vi "FAR_IR_CM_to_NEAR_IR_NM.vi"(11 "Far IR / cm-1":dbl) -> (3 "Near IR / nm":dbl format="%#_6f")   [LabVIEW 2020]
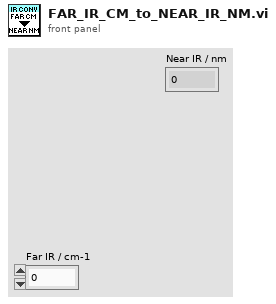
[diagram p1: front panel]
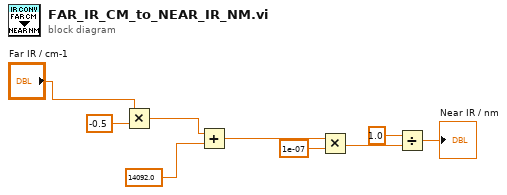
[diagram p0: block diagram]
diagram:
  n1 = Multiply(x="Far IR / cm-1", y=-0.5) -> (x*y=w3:dbl)
  n2 = Add(x=w3, y=14092.0) -> (x+y=w8:dbl)
  n3 = Multiply(x=w8, y=1e-07) -> (x*y=w6:dbl)
  n4 = Divide(x=1.0, y=w6) -> (x/y=→"Near IR / nm":dbl)
